vi "Get Temperature.vi"(6 "Channel":i32, 8 "error in (no error)":errorcluster, 11 "instrument.Cryostation in":refnum<class "instrument.Cryostation.lvclass">) -> (0 "error out":errorcluster, 1 "Status":string, 2 "Temperature (K)":dbl, 3 "instrument.Cryostation out":refnum<class "instrument.Cryostation.lvclass">, 4 "Finished?":bool)   [LabVIEW 2019, in "instrument.Cryostation.lvclass"]
uses:
  instrument.Cryostation.lvclass
  C:/Program Files (x86)/National Instruments/LabVIEW 2019/user.lib/LevyLab/Levylab Instruments/SMOs/Instrument/Instrument.lvclass
  Typedefs/Cryostation.Commands--enum.ctl
  <userlib>/LevyLab/Levylab Instruments/SMOs/Instrument/Instrument.lvclass/Instrument.ctl
  b940bc90-ff77-425f-b322-deebe51aed3a.vi
  b940bc90-ff77-425f-b322-deebe51aed3a.vi/7ce6df9d-6737-4512-875d-c36e9176cc00.vi
  b940bc90-ff77-425f-b322-deebe51aed3a.vi/7ce6df9d-6737-4512-875d-c36e9176cc00.vi/f9a256e5-9871-4fc5-ac09-50ba22286f58.vi
  b940bc90-ff77-425f-b322-deebe51aed3a.vi/7ce6df9d-6737-4512-875d-c36e9176cc00.vi/9affe925-a5a6-4726-a27a-228acb9e2e5a.vi
  <userlib>/LevyLab/Levylab Instruments/SMOs/Instrument/API/Send and Receive.vi
  b940bc90-ff77-425f-b322-deebe51aed3a.vi/7ce6df9d-6737-4512-875d-c36e9176cc00.vi/9affe925-a5a6-4726-a27a-228acb9e2e5a.vi/d8514108-0e3f-44e2-8137-1e1271062cd0.vi
  b940bc90-ff77-425f-b322-deebe51aed3a.vi/7ce6df9d-6737-4512-875d-c36e9176cc00.vi/9affe925-a5a6-4726-a27a-228acb9e2e5a.vi/cb795813-4d02-434e-ad7d-4b2361b5af5b.vi
  b940bc90-ff77-425f-b322-deebe51aed3a.vi/7ce6df9d-6737-4512-875d-c36e9176cc00.vi/9affe925-a5a6-4726-a27a-228acb9e2e5a.vi/861afb43-15b2-4066-8761-e2f0e39015b5.vi
  <userlib>/LevyLab/Levylab Instruments/SMOs/RemoteControl/API/Send and Receive.vi
  <vilib>/JDP Science/JSONtext/JSON text to Variant.vi
  <vilib>/JDP Science/JSONtext/LVClass Serializer/JSONtext LVClass Serializer.lvclass
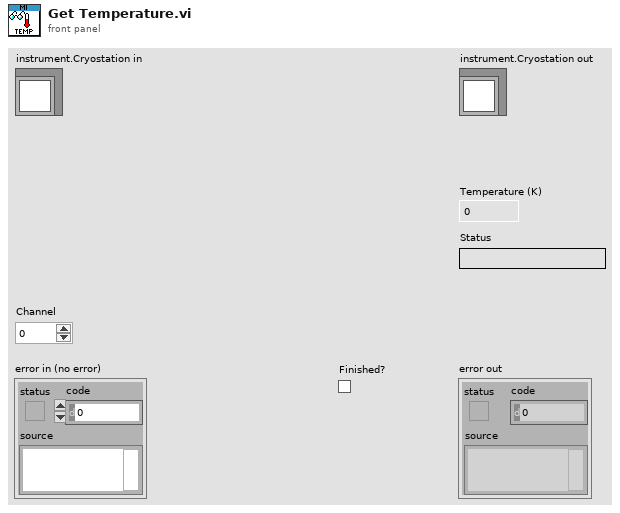
[diagram p1: front panel]
types:
  T1 = typedef "instrument.Cryostation.lvclass/Cryostation.Commands--enum.ctl" = enum16{"Get Temperature"}
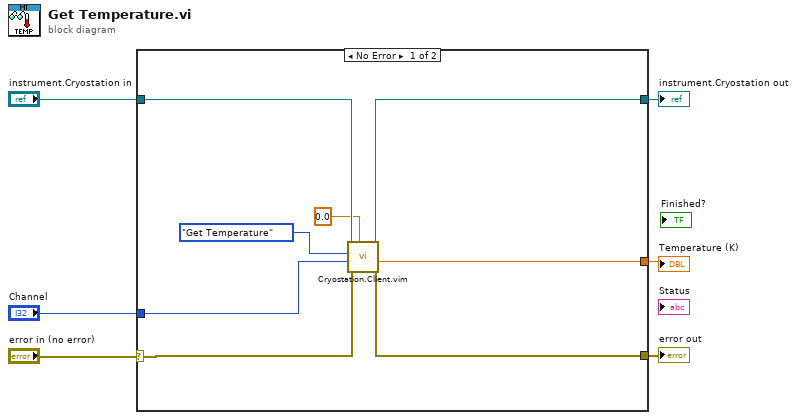
[diagram p0: block diagram]
diagram:
  n1 = case shown="No Error" "error in (no error)" {
    selector: "error in (no error)" -> [w11 w16]
    tunnel: [w14 _] -> w6
    tunnel: [w9 w16] -> w5
    tunnel: [w13 w15] -> w4
    tunnel: "instrument.Cryostation in" -> [w12 w15]
    tunnel: "Channel" -> [w10 _]
    frame No Error {
      n2 = call "Cryostation.Client.vim"("Data Out type"=0.0 ("Temperature (K)"), "error in (no error)"=w11, "Data"=w10, "Command"=Cryostation.Commands--enum."Get Temperature", "instrument.Cryostation in"=w12) -> ("error out"=w9:errorcluster, "Data out"=w14:dbl, "instrument.Cryostation out"=w13:refnum<class "instrument.Cryostation.lvclass">)  [unwired: 3 in, 1 out]
    }
    frame Error {
    }
  }
  "error out" <- w5
  "instrument.Cryostation out" <- w4
  "Temperature (K)" <- w6
